vi "Create.vi"(8 "error in (no error)":errorcluster, 11 "Plugins":refnum<class "Plugin.lvclass">[](array[class])) -> (0 "error out":errorcluster, 3 "Buffers Map out":refnum<class "Buffers Map.lvclass">)   [LabVIEW 2017, in "DSF Core.lvlib" / "Buffers Map.lvclass"]
uses:
  Buffers Map.lvclass
  Plugin/Plugin.lvclass
  Plugin.ctl
  Buffers/Buffers.lvclass
  Group.ctl
  Transfer/Transfer.lvclass
  Buffers Map.lvclass/Buffers Map.ctl
  Transfer Group/Transfer Group.lvclass
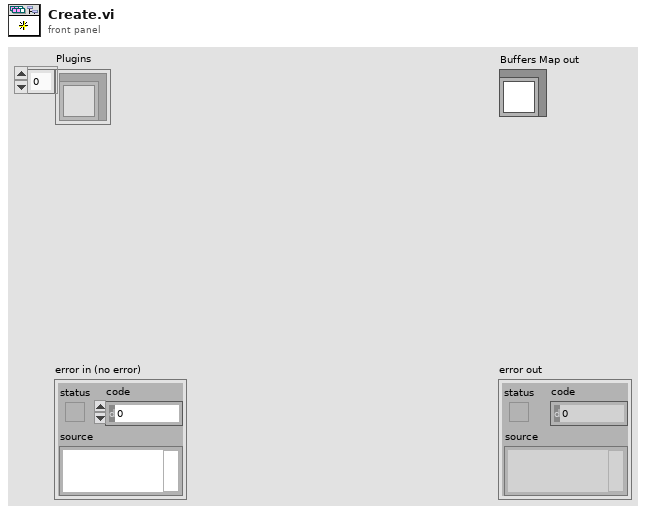
[diagram p1: front panel]
types:
  T1 = typedef "DSF Core.lvlib/Buffers Map.lvclass/Plugin.ctl" = cluster{"Plugin Buffers":refnum<class "Buffers.lvclass">, "Groups":T2[]}
  T2 = typedef "DSF Core.lvlib/Buffers Map.lvclass/Group.ctl" = cluster{"Group Buffers":refnum<class "Buffers.lvclass">, "Transfers":refnum<class "Transfer.lvclass">[]}
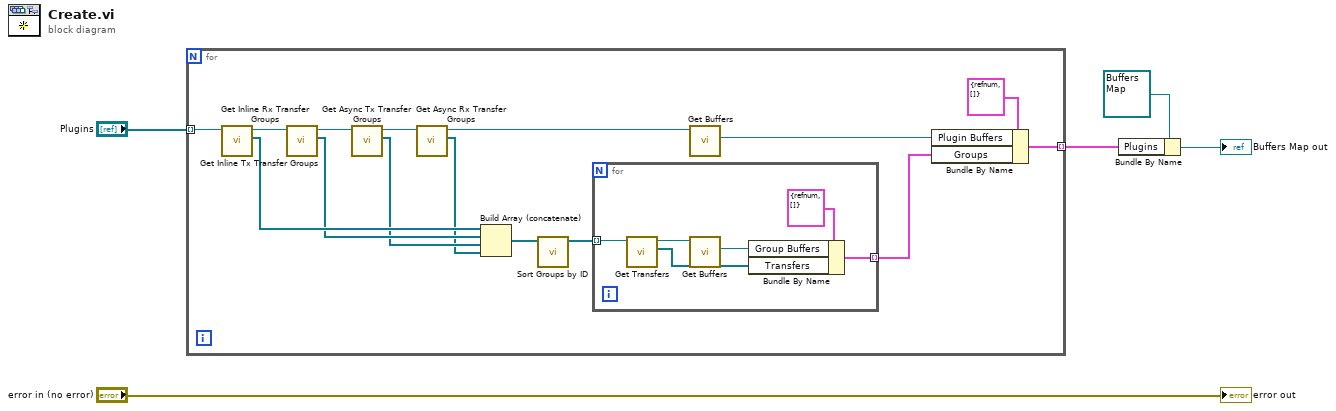
[diagram p0: block diagram]
diagram:
  n1 = for {
    tunnel: "Plugins" -> [w17] mode=indexing
    tunnel: [w19] -> w1 mode=indexing
    n2 = call "Get Inline Rx Transfer Groups.vi"("Plugin in"=w17) -> ("Inline Rx Transfer Groups"=w13:refnum<class "Transfer Group.lvclass">[], "Plugin out"=w16:refnum<class "Plugin.lvclass">)  [unwired: 9 in]
    n3 = call "Get Inline Tx Transfer Groups.vi"("Plugin in"=w16) -> ("Inline Tx Transfer Groups"=w12:refnum<class "Transfer Group.lvclass">[], "Plugin out"=w15:refnum<class "Plugin.lvclass">)  [unwired: 9 in]
    n4 = call "Get Async Tx Transfer Groups.vi"("Plugin in"=w15) -> ("Async Tx Transfer Groups"=w11:refnum<class "Transfer Group.lvclass">[], "Plugin out"=w14:refnum<class "Plugin.lvclass">)  [unwired: 9 in]
    n5 = call "Get Async Rx Transfer Groups.vi"("Plugin in"=w14) -> ("Async Rx Transfer Groups"=w8:refnum<class "Transfer Group.lvclass">[], "Plugin out"=w9:refnum<class "Plugin.lvclass">)  [unwired: 9 in]
    n6 = Build Array (concatenate)(w13, w12, w11, w8) -> (w10:refnum<class "Transfer Group.lvclass">[])
    n7 = call "Sort Groups by ID.vi"("Transfers Groups in"=w10) -> ("ID-sorted Transfers Groups out"=w7:refnum<class "Transfer Group.lvclass">[])  [unwired: 9 in, 1 out]
    n8 = for {
      tunnel: w7 -> [w23] mode=indexing
      tunnel: [w24] -> w6 mode=indexing
      n9 = call "Get Transfers.vi"("Transfer Group in"=w23) -> ("Transfers"=w21:refnum<class "Transfer.lvclass">[], "Transfer Group out"=w22:refnum<class "Transfer Group.lvclass">)  [unwired: 9 in]
      n10 = call "Get Buffers.vi"("Transfer Group in"=w22) -> ("Buffers"=w25:refnum<class "Buffers.lvclass">)  [unwired: 9 in, 1 out]
      n11 = Bundle By Name(cluster=T2 {"Group Buffers"=refnum, "Transfers"=[]} ("Group"), "Group Buffers"=w25, "Transfers"=w21) -> (w24:T2)
    }
    n12 = call "Get Buffers.vi"("Plugin in"=w9) -> ("Buffers"=w18:refnum<class "Buffers.lvclass">)  [unwired: 9 in, 1 out]
    n13 = Bundle By Name(cluster=T1 {"Plugin Buffers"=refnum, "Groups"=[]} ("Plugin"), "Plugin Buffers"=w18, "Groups"=w6) -> (w19:T1)
  }
  n14 = Bundle By Name(cluster=refnum<class "Buffers Map.lvclass"> refnum ("Buffers Map in"), "Plugins"=w1) -> (→"Buffers Map out":refnum<class "Buffers Map.lvclass">)
  "error out" <- "error in (no error)"
